vi "Get Component Path.vi"(8 "Error In":errorcluster, 11 "Configuration":T1) -> (0 "Error Out":errorcluster, 2 "Component Install Paths":path[](array[path]), 3 "Configuration":T1)   [LabVIEW 2011, in "LVH-Build-Tools.lvlib"]
uses:
  <vilib>/LabVIEW Hacker/Build Tools/LVH-Build-Tools.lvlib
  Type Defs/Configuration.ctl
  Type Defs/Install Configuration.ctl
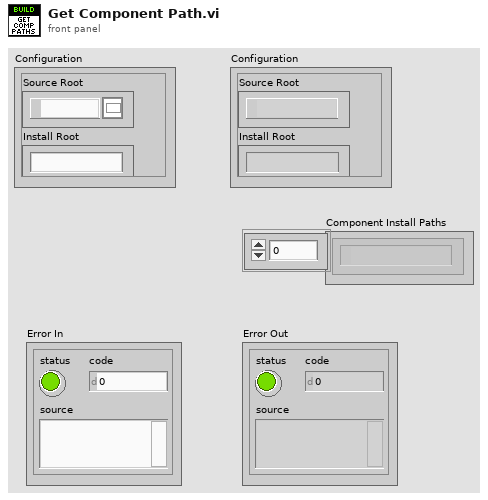
[diagram p1: front panel]
types:
  T1 = typedef "LVH-Build-Tools.lvlib/Configuration.ctl" = cluster{"Source Root":path, "Install Root":string, "Components":string[], "Ignore":string[], "Config Files":path[], "LV Directories":path[], "Install Paths":T2}
  T2 = typedef "LVH-Build-Tools.lvlib/Install Configuration.ctl" = cluster{"LabVIEW Directory":path, "Project Source Config":path}
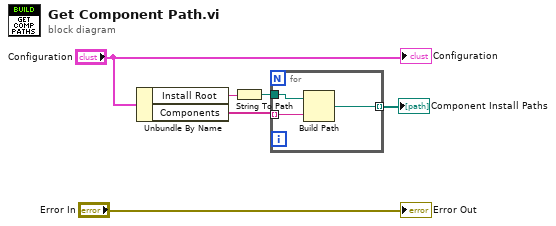
[diagram p0: block diagram]
diagram:
  n1 = Unbundle By Name("Configuration") -> ("Install Root"=w3:string, "Components"=w5:string[])
  n2 = String To Path(string=w3) -> (path=w2:path)
  n3 = for {
    tunnel: w5 -> [w9] mode=indexing
    tunnel: w2 -> [w8]
    tunnel: [w7] -> w1 mode=indexing
    n4 = Build Path(base path=w8, name or relative path=w9) -> (appended path=w7:path)
  }
  "Component Install Paths" <- w1
  "Error Out" <- "Error In"
  "Configuration" <- "Configuration"
